vi "GetInitialDirection.vi"(8 "error in (no error)":errorcluster, 11 "reference in":refnum<class "Ball.lvclass">) -> (0 "error out":errorcluster, 2 "InitialDirection":csg, 3 "reference out":refnum<class "Ball.lvclass">)   [LabVIEW 2010, in "Labricks.lvlib" / "Ball.lvclass"]
doc: "Accesses the initial direction of the ball."
uses:
  Ball.lvclass
  Ball.lvclass/Ball.ctl
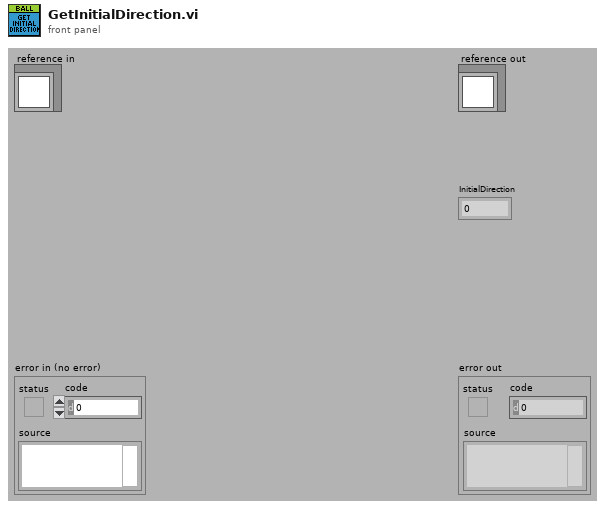
[diagram p1: front panel]
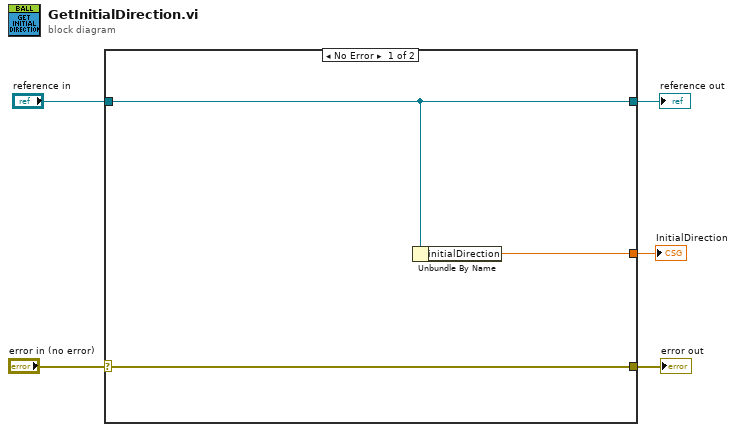
[diagram p0: block diagram]
diagram:
  n1 = case shown="No Error" "error in (no error)" {
    selector: "error in (no error)" -> [w6 w10]
    tunnel: [w6 w10] -> w4
    tunnel: [w8 w9] -> w2
    tunnel: "reference in" -> [w8 w9]
    tunnel: [w7 _] -> w1
    frame No Error {
      n2 = Unbundle By Name(w8) -> ("initialDirection"=w7:csg)
    }
    frame Error {
    }
  }
  "error out" <- w4
  "reference out" <- w2
  "InitialDirection" <- w1
